vi "Display Info.vi"(7 "Layout ref":refnum<vi>, 8 "error in (no error)":errorcluster, 9 "Modify (F) /Add [T]":bool, 10 "Names in use":string[](array[string]), 11 "DDS in":refnum<class "DDS.lvclass">) -> (0 "error out":errorcluster, 1 "Names in use out":string[](array[string]), 2 "Changes Made?":bool, 3 "DDS out":refnum<class "DDS.lvclass">)   [LabVIEW 2013, in "DDS.lvclass"]
uses:
  DDS.lvclass
  TypeDefs/DigitalColumnAppearCluster.ctl
  TypeDefs/ColumnAppearCluster.ctl
  DDS.lvclass/DDS.ctl
  ColumnVIs/Column/Column.lvclass
panel:
  out "Col. Appear. Labels":string[](array[string])
  in  "Column appearance":T1[](array[typedef])
  in  "Sweep Dir. Appearance":T2={"Column Name"="", "Width"=18, "Bkgd"=[1985280, 6618880, 14090026], "Text"=[16448250, 0, 0]}
  in  "Cancel":bool
  in  "Device Description":string
  in  "DDS config":T3={"PB trig / Sequence"=FALSE, "Sweeps"=FALSE, "Amp Lock"=FALSE, "Master Trig. Line"=4, "USB Chan. name"=""}
  in  "Done":bool
  in  "Name":string
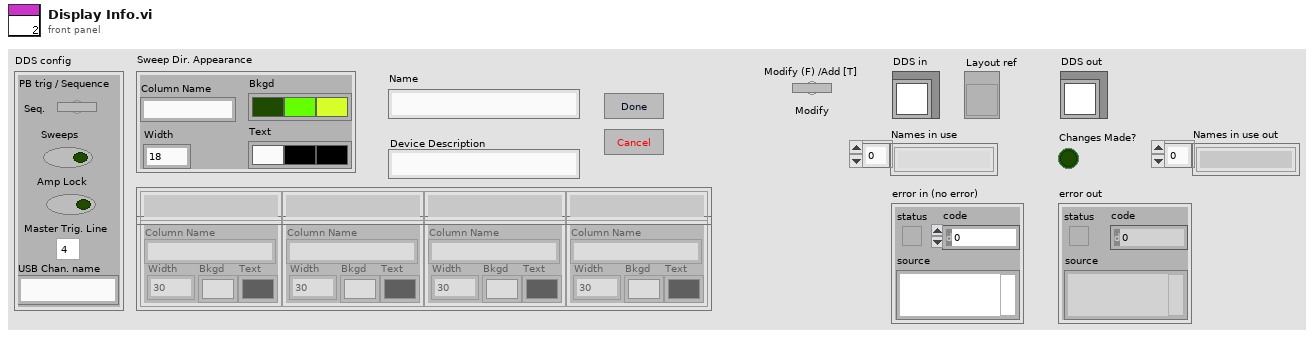
[diagram p1: front panel]
types:
  T1 = typedef "ColumnAppearCluster.ctl" = cluster{"Column Name":string, "Width":u32, "Bkgd":u32[], "Text":u32[]}
  T2 = typedef "DigitalColumnAppearCluster.ctl" = cluster{"Column Name":string, "Width":u32, "Bkgd":u32[], "Text":u32[]}
  T3 = cluster{"PB trig / Sequence":bool, "Sweeps":bool, "Amp Lock":bool, "Master Trig. Line":u16, "USB Chan. name":string}
  T4 = enum8{"Enabled", "Disabled", "Disabled and Grayed Out"}
  T5 = cluster{"Sweeps":bool, "PB trig / Sequence":bool, "Amp Lock":bool, "Firmware Ver":dbl}
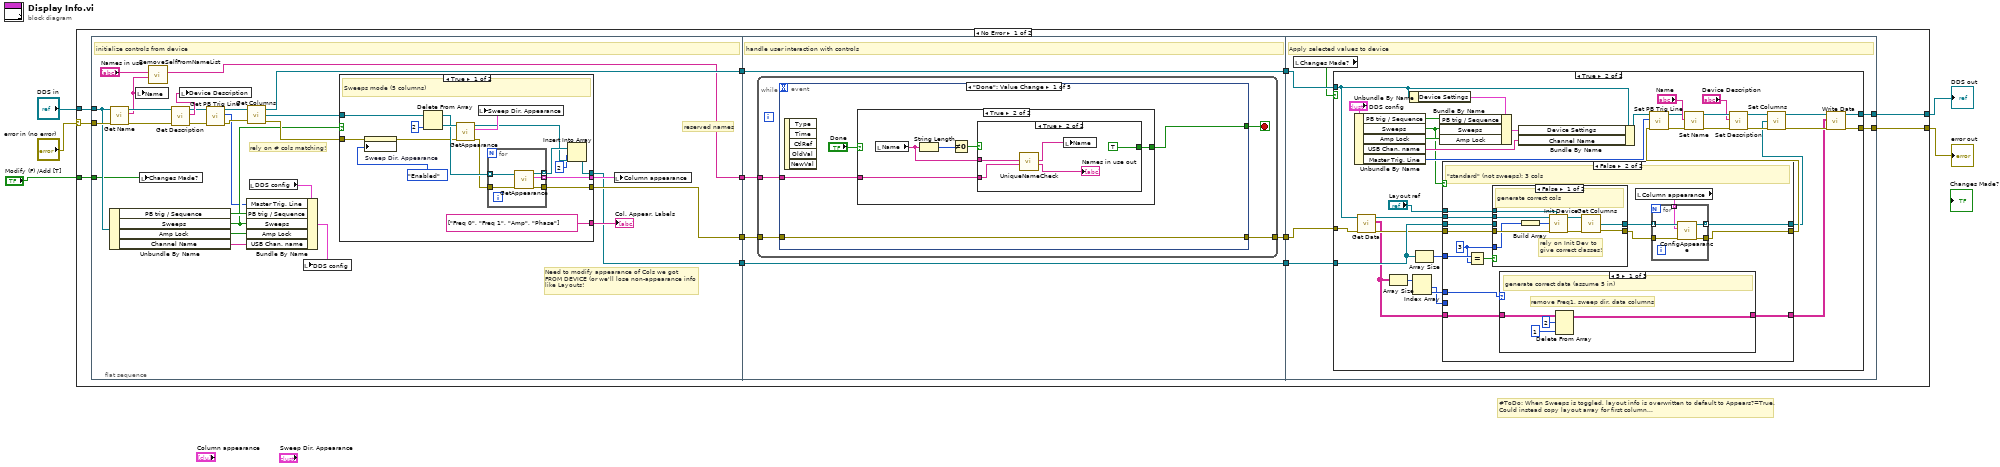
[diagram p0: block diagram]
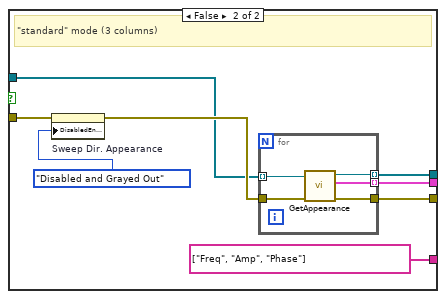
[diagram p2: hidden frame]
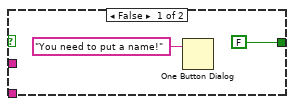
[diagram p4: hidden frame]
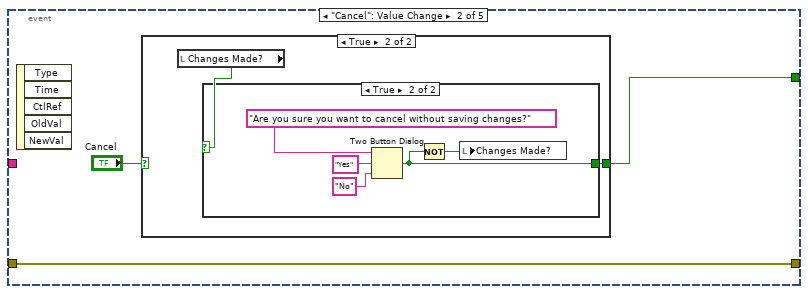
[diagram p5: hidden frame]
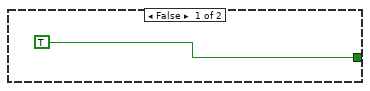
[diagram p7: hidden frame]
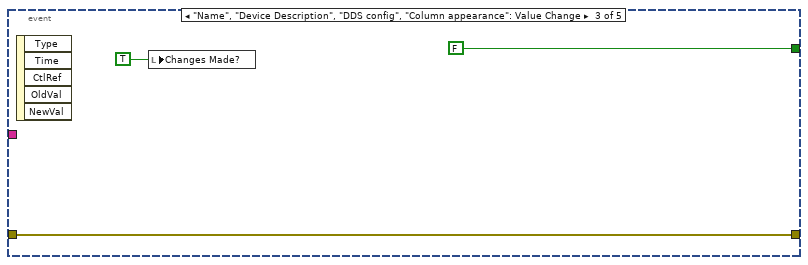
[diagram p8: hidden frame]
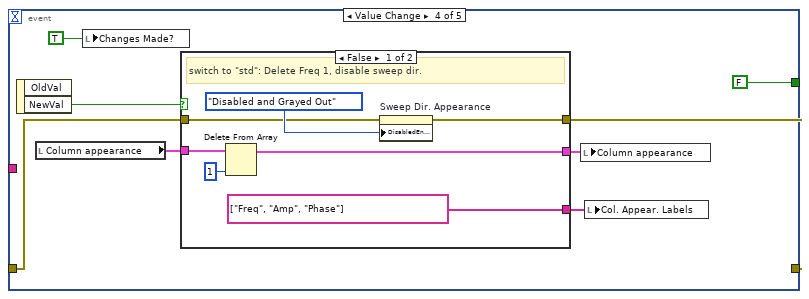
[diagram p9: hidden frame]
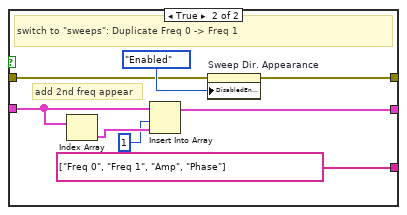
[diagram p10: hidden frame]
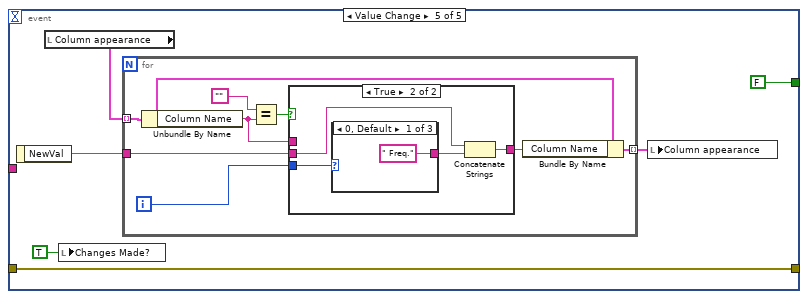
[diagram p11: hidden frame]
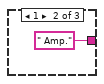
[diagram p13: hidden frame]
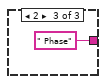
[diagram p14: hidden frame]
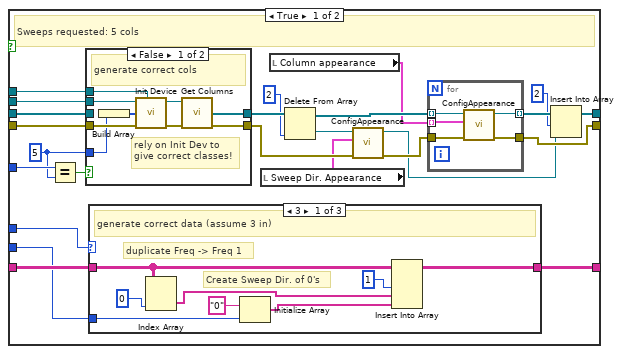
[diagram p16: hidden frame]
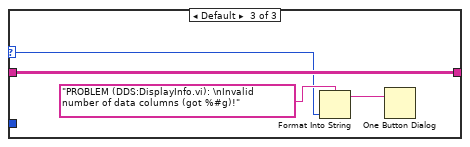
[diagram p18: hidden frame]
diagram:
  # "#ToDo: When Sweeps is toggled, layout info is overwritten to default to Appears?=True.\nCould instead copy layout array for first column..."
  n1 = case shown="No Error" "error in (no error)" {
    selector: "error in (no error)" -> [w14 w302]
    tunnel: [w11 w302] -> w4
    tunnel: "DDS in" -> [w8 w301]
    tunnel: [w17 w301] -> w2
    tunnel: "Modify (F) /Add [T]" -> [w7 _]
    frame No Error {
      n2 = flat-sequence {
        tunnel: [w43] -> w16
        tunnel: w14 -> [w30]
        tunnel: [w29] -> w13
        tunnel: [w28] -> w10
        tunnel: w8 -> [w22]
        tunnel: w7 -> [w21]
        tunnel: [w18] -> w6
        tunnel: w16 -> [w83]
        tunnel: [w83] -> w15
        tunnel: w13 -> [w82]
        tunnel: [w81] -> w12
        tunnel: w10 -> [w80]
        tunnel: [w80] -> w9
        tunnel: w6 -> [w79]
        tunnel: [w170] -> w17
        tunnel: w15 -> [w169]
        tunnel: w12 -> [w165]
        tunnel: [w167] -> w11
        tunnel: w9 -> [w166]
        frame #0 {
          # "reserved names"
          # "Need to modify appearance of Cols we got\nFROM DEVICE (or we'll lose non-appearance info\nlike Layouts!"
          # "rely on # cols matching!"
          # "initialize controls from device"
          n3 = Unbundle By Name(w22) -> ("PB trig / Sequence"=w27:bool, "Sweeps"=w26:bool, "Amp Lock"=w25:bool, "Channel Name"=w40:string)
          n4 = call-dynamic "Get Name.vi"("error in (no error)"=w30, "Device in"=w22) -> ("error out"=w37:errorcluster, "Name"=w19:string, "Device out"=w39:refnum<class "DDS.lvclass">)  [unwired: 7 in]
          n5 = local write "Name"(w19) -> ()
          n6 = local write "Changes Made?"(w21) -> ()
          n7 = call "RemoveSelfFromNameList.vi"("self Name"=w19, "Names in use"="Names in use") -> ("Reserved Names"=w18:string[])  [unwired: 9 in]
          n8 = call-dynamic "Get Description.vi"("error in (no error)"=w37, "Device in"=w39) -> ("error out"=w36:errorcluster, "Device Description"=w44:string, "Device out"=w38:refnum<class "DDS.lvclass">)  [unwired: 7 in]
          n9 = local write "Device Description"(w44) -> ()
          n10 = call-dynamic "Get PB Trig Line.vi"("error in (no error)"=w36, "Device in"=w38) -> ("error out"=w34:errorcluster, "PB Trigger Line"=w24:u16, "Device out"=w35:refnum<class "DDS.lvclass">)  [unwired: 7 in]
          n11 = call-dynamic "Get Columns.vi"("Device in"=w35, "error in (no error)"=w34) -> ("Device out"=w43:refnum<class "DDS.lvclass">, "Columns"=w23:refnum<class "Column.lvclass">[], "error out"=w33:errorcluster)
          n12 = local read "DDS config"() -> (w42:T3)
          n13 = Bundle By Name(cluster=w42, "Master Trig. Line"=w24, "PB trig / Sequence"=w27, "Sweeps"=w26, "Amp Lock"=w25, "USB Chan. name"=w40) -> (w41:T3)
          n14 = local write "DDS config"(w41) -> ()
          n15 = case shown="True" w26 {
            tunnel: w33 -> [w52 w71]
            tunnel: w23 -> [w57 w68]
            tunnel: [string[] ["Freq 0", "Freq 1", "Amp", "Phase"] ("Col. Appear. Labels") string[] ["Freq", "Amp", "Phase"] ("Col. Appear. Labels")] -> w32
            tunnel: [w53 w72] -> w31
            tunnel: [w49 w67] -> w29
            tunnel: [w47 w66] -> w28
            frame True {
              # "Sweeps mode (5 columns)"
              n16 = property on="Sweep Dir. Appearance" class="Clust (strict)"(error in=w52, "DisabledEnum"=T4."Enabled" ("Disabled")) -> (error out=w51:errorcluster)  [unwired: 1 in, 1 out]
              n17 = Delete From Array "Delete From Array"(array=w57, index=2) -> (deleted portion=w59:refnum<class "Column.lvclass">, array with subset deleted=w56:refnum<class "Column.lvclass">[])  [unwired: 1 in]
              n18 = call "GetAppearance.vi"("error in (no error)"=w51, "Column in"=w59) -> ("error out"=w55:errorcluster, "Column Appearance"=w58:T1, "Column out"=w46:refnum<class "Column.lvclass">)  [unwired: 7 in]
              n19 = local write "Sweep Dir. Appearance"(w58) -> ()
              n20 = for {
                tunnel: w56 -> [w65] mode=indexing
                tunnel: w55 -> [w64]
                tunnel: [w63] -> w53 mode=indexing
                tunnel: [w62] -> w49
                tunnel: [w61] -> w48 mode=indexing
                n21 = call "GetAppearance.vi"("error in (no error)"=w64, "Column in"=w65) -> ("error out"=w62:errorcluster, "Column Appearance"=w63:T1, "Column out"=w61:refnum<class "Column.lvclass">)  [unwired: 7 in]
              }
              n22 = Insert Into Array(array=w48, index=2, new element=w46) -> (w47:refnum<class "Column.lvclass">[])
            }
            frame False {
              # "\"standard\" mode (3 columns)"
              n23 = property on="Sweep Dir. Appearance" class="Clust (strict)"(error in=w71, "DisabledEnum"=T4."Disabled and Grayed Out" ("Disabled")) -> (error out=w69:errorcluster)  [unwired: 1 in, 1 out]
              n24 = for {
                tunnel: w68 -> [w78] mode=indexing
                tunnel: w69 -> [w77]
                tunnel: [w76] -> w72 mode=indexing
                tunnel: [w75] -> w67
                tunnel: [w74] -> w66 mode=indexing
                n25 = call "GetAppearance.vi"("error in (no error)"=w77, "Column in"=w78) -> ("error out"=w75:errorcluster, "Column Appearance"=w76:T1, "Column out"=w74:refnum<class "Column.lvclass">)  [unwired: 7 in]
              }
            }
          }
          "Col. Appear. Labels" <- w32
          n26 = local write "Column appearance"(w31) -> ()
        }
        frame #1 {
          # "handle user interaction with controls"
          n27 = while {
            tunnel: w82 -> [w86]
            tunnel: [w85] -> w81
            tunnel: w79 -> [w84]
            stop <- w87 stop-if-true
            n28 = event shown="[0] \"Done\": Value Change" {
              selector: _ -> [_ _ _ _ _]
              dyn-events: _ -> [_ _ _ _ _]
              timeout: _ -> [_ _ _ _ _]
              tunnel: [w90 w106 FALSE ("T button?") FALSE ("T button?") FALSE ("T button?")] -> w87
              tunnel: w86 -> [w89 w105 w117 w121 w143]
              tunnel: [w89 w105 w117 w120 w143] -> w85
              tunnel: w84 -> [w88 _ _ _ _]
              event "Done": Value Change {
                n29 = event-data() -> ()  [unwired: 1 in, 5 out]
                n30 = case shown="True" "Done" {
                  selector: "Done" -> [w92 _]
                  tunnel: [w92 w95] -> w90
                  tunnel: w88 -> [_ w93]
                  frame False {
                  }
                  frame True {
                    n31 = local read "Name"() -> (w94:string)
                    n32 = String Length(string=w94) -> (length=w97:i32)
                    n33 = Not Equal To 0?(x=w97) -> (x != 0?=w96:bool)
                    n34 = case shown="True" w96 {
                      tunnel: [FALSE TRUE] -> w95
                      tunnel: w94 -> [_ w103]
                      tunnel: w93 -> [_ w102]
                      frame False {
                        n35 = One Button Dialog(message="You need to put a name!") -> ()  [unwired: 1 in, 1 out]
                      }
                      frame True {
                        n36 = call "UniqueNameCheck.vi"("Names in use"=w102, "Device Name"=w103) -> ("Names in use out"=→"Names in use out":string[], "Unique name"=w101:string)  [unwired: 8 in]
                        n37 = local write "Name"(w101) -> ()
                      }
                    }
                  }
                }
              }
              event "Cancel": Value Change {
                n38 = event-data() -> ()  [unwired: 1 in, 5 out]
                n39 = case shown="True" "Cancel" {
                  selector: "Cancel" -> [w108 _]
                  tunnel: [w108 w110] -> w106
                  frame False {
                  }
                  frame True {
                    n40 = local read "Changes Made?"() -> (w109:bool)
                    n41 = case shown="True" w109 {
                      tunnel: [TRUE w113] -> w110
                      frame False {
                      }
                      frame True {
                        n42 = Two Button Dialog(message="Are you sure you want to cancel without saving changes?", 1:"No", 2:"Yes") -> (T button?=w113:bool)
                        n43 = Not(x=w113) -> (.not. x?=w112:bool)
                        n44 = local write "Changes Made?"(w112) -> ()
                      }
                    }
                  }
                }
              }
              event "Name", "Device Description", "DDS config", "Column appearance": Value Change {
                n45 = event-data() -> ()  [unwired: 1 in, 5 out]
                n46 = local write "Changes Made?"(TRUE) -> ()
              }
              event "DDS config.Sweeps": Value Change {
                n47 = event-data() -> ("NewVal"=w126:bool)  [unwired: 1 in, 1 out]
                n48 = local read "Column appearance"() -> (w124:T1[])
                n49 = local write "Changes Made?"(TRUE ("Changes Made?")) -> ()
                n50 = case shown="False" w126 {
                  tunnel: [string[] ["Freq", "Amp", "Phase"] ("Col. Appear. Labels") string[] ["Freq 0", "Freq 1", "Amp", "Phase"] ("Col. Appear. Labels")] -> w125
                  tunnel: w124 -> [w132 w139]
                  tunnel: [w130 w140] -> w123
                  tunnel: w121 -> [w129 w135]
                  tunnel: [w128 w136] -> w120
                  frame False {
                    # "switch to \"std\": Delete Freq 1, disable sweep dir."
                    n51 = Delete From Array "Delete From Array"(array=w132, index=1) -> (array with subset deleted=w130:T1[])  [unwired: 1 in, 1 out]
                    n52 = property on="Sweep Dir. Appearance" class="Clust (strict)"(error in=w129, "DisabledEnum"=T4."Disabled and Grayed Out" ("Disabled")) -> (error out=w128:errorcluster)  [unwired: 1 in, 1 out]
                  }
                  frame True {
                    # "add 2nd freq appear"
                    # "switch to \"sweeps\": Duplicate Freq 0 -> Freq 1"
                    n53 = Index Array(array=w139) -> (element=w138:T1)  [unwired: 1 in]
                    n54 = Insert Into Array "Insert Into Array"(array=w139, index=1, new element=w138) -> (w140:T1[])
                    n55 = property on="Sweep Dir. Appearance" class="Clust (strict)"(error in=w135, "DisabledEnum"=T4."Enabled" ("Disabled")) -> (error out=w136:errorcluster)  [unwired: 1 in, 1 out]
                  }
                }
                n56 = local write "Column appearance"(w123) -> ()
                n57 = local write "Col. Appear. Labels"(w125) -> ()
              }
              event "DDS config.USB Chan. name": Value Change {
                n58 = event-data() -> ("NewVal"=w147:string)  [unwired: 1 in]
                n59 = local read "Column appearance"() -> (w145:T1[])
                n60 = local write "Changes Made?"(TRUE) -> ()
                n61 = for {
                  tunnel: w145 -> [w152] mode=indexing
                  tunnel: [w153] -> w144 mode=indexing
                  tunnel: w147 -> [w151]
                  i -> [w155]
                  n62 = Unbundle By Name(w152) -> ("Column Name"=w149:string)
                  n63 = Equal?(x="", y=w149) -> (x = y?=w154:bool)
                  n64 = case shown="True" w154 {
                    tunnel: w151 -> [_ w158]
                    tunnel: [w157 w159] -> w156
                    tunnel: w155 -> [_ w161]
                    tunnel: w149 -> [w157 _]
                    frame False {
                    }
                    frame True {
                      n65 = case shown="0, Default" w161 {
                        tunnel: [" Freq." " Amp." " Phase"] -> w160
                        frame 0, Default {
                        }
                        frame 1 {
                        }
                        frame 2 {
                        }
                      }
                      n66 = Concatenate Strings(w158, w160) -> (w159:string)
                    }
                  }
                  n67 = Bundle By Name(cluster=w152, "Column Name"=w156) -> (w153:T1)
                }
                n68 = local write "Column appearance"(w144) -> ()
              }
            }
          }
        }
        frame #2 {
          # "Apply selected values to device"
          n69 = local read "Changes Made?"() -> (w168:bool)
          n70 = case shown="True" w168 {
            tunnel: [w172 w178] -> w170
            tunnel: w169 -> [w172 w185]
            tunnel: [w171 w176] -> w167
            tunnel: w166 -> [_ w189]
            tunnel: w165 -> [w171 w184]
            frame False {
            }
            frame True {
              n71 = Unbundle By Name("DDS config") -> ("PB trig / Sequence"=w202:bool, "Sweeps"=w192:bool, "Amp Lock"=w201:bool, "USB Chan. name"=w199:string, "Master Trig. Line"=w198:u16)
              n72 = call-dynamic "Get Data.vi"("error in (no error)"=w184, "Device in"=w185) -> ("error out"=w182:errorcluster, "Table Indicator"=w181:string[][], "Device out"=w183:refnum<class "DDS.lvclass">)  [unwired: 6 in]
              n73 = Array Size(array=w181) -> (size(s)=w180:i32[])
              n74 = Unbundle By Name(w185) -> ("Device Settings"=w203:T5)
              n75 = Index Array(array=w180) -> (element #1=w173:i32, element #2=w174:i32)  [unwired: 2 in]
              n76 = Array Size(array=w189) -> (size(s)=w191:i32)
              n77 = Bundle By Name(cluster=w203, "PB trig / Sequence"=w202, "Sweeps"=w192, "Amp Lock"=w201) -> (w200:T5)
              n78 = case shown="False" w192 {
                tunnel: w191 -> [w231 w275]
                tunnel: w189 -> [w229 w274]
                tunnel: [w217 w271] -> w188
                tunnel: [w220 w272] -> w187
                tunnel: "Layout ref" -> [w215 w267]
                tunnel: w183 -> [w214 w266]
                tunnel: w182 -> [w213 w265]
                tunnel: w181 -> [w211 w264]
                tunnel: w174 -> [w209 w262]
                tunnel: [w212 w263] -> w175
                tunnel: w173 -> [w210 _]
                frame True {
                  w208 = 5 ("index")
                  # "Sweeps requested: 5 cols"
                  n79 = Equal?(x=w231, y=w208) -> (x = y?=w230:bool)
                  n80 = case shown="False" w230 {
                    tunnel: w214 -> [w258 _]
                    tunnel: [w255 w260] -> w228
                    tunnel: w229 -> [_ w260]
                    tunnel: [w254 w259] -> w223
                    tunnel: w213 -> [w253 w259]
                    tunnel: w215 -> [w252 _]
                    tunnel: w208 -> [w250 _]
                    frame False {
                      # "rely on Init Dev to \ngive correct classes!"
                      # "generate correct cols"
                      n81 = Build Array(w250) -> (w251:i32[])
                      n82 = call-dynamic "Init Device.vi"("Layout Ref"=w252, "error in (no error)"=w253, "Chan# Array"=w251, "DDS in"=w258) -> ("error out"=w256:errorcluster, "DDS out"=w257:refnum<class "DDS.lvclass">)  [unwired: 6 in]
                      n83 = call-dynamic "Get Columns.vi"("Device in"=w257, "error in (no error)"=w256) -> ("Columns"=w255:refnum<class "Column.lvclass">[], "error out"=w254:errorcluster)  [unwired: 1 out]
                    }
                    frame True {
                      # "correct # cols"
                    }
                  }
                  n84 = case shown="3" w209 {
                    selector: w209 -> [_ _ w242]
                    tunnel: [w238 w240 w244] -> w212
                    tunnel: w211 -> [w237 w240 w244]
                    tunnel: w210 -> [w234 _ _]
                    frame 3 {
                      # "Create Sweep Dir. of 0's"
                      # "duplicate Freq -> Freq 1"
                      # "generate correct data (assume 3 in)"
                      n85 = Index Array(array=w237, index (col)=0 ("disabled index (col)")) -> (element=w232:string[])  [unwired: 1 in]
                      n86 = Initialize Array("0", w234) -> (w233:string[])
                      n87 = Insert Into Array(array=w237, index (col)=1 ("disabled index (col)"), new element #1=w232, new element #2=w233) -> (w238:string[][])  [unwired: 1 in]
                    }
                    frame 0, 5 {
                      # "If length is 0, Default Data will take care within Add device."
                      # "correct data size"
                    }
                    frame Default {
                      n88 = Format Into String(format string="PROBLEM (DDS:DisplayInfo.vi): \nInvalid number of data columns (got %#g)!" ("message"), w242) -> (resulting string=w241:string)  [unwired: 2 in, 1 out]
                      n89 = One Button Dialog(message=w241) -> ()  [unwired: 1 in, 1 out]
                    }
                  }
                  n90 = local read "Sweep Dir. Appearance"() -> (w218:T2)
                  n91 = local read "Column appearance"() -> (w225:T1[])
                  n92 = Delete From Array(array=w228, index=2) -> (deleted portion=w224:refnum<class "Column.lvclass">, array with subset deleted=w226:refnum<class "Column.lvclass">[])  [unwired: 1 in]
                  n93 = call "ConfigAppearance.vi"("error in (no error)"=w223, "Column Appearance"=w218, "Column in"=w224) -> ("error out"=w222:errorcluster, "Column out"=w216:refnum<class "Column.lvclass">)  [unwired: 7 in]
                  n94 = for {
                    tunnel: w226 -> [w249] mode=indexing
                    tunnel: [w248] -> w221 mode=indexing
                    tunnel: [w247] -> w217
                    tunnel: w222 -> [w246]
                    tunnel: w225 -> [w245] mode=indexing
                    n95 = call "ConfigAppearance.vi"("error in (no error)"=w246, "Column Appearance"=w245, "Column in"=w249) -> ("error out"=w247:errorcluster, "Column out"=w248:refnum<class "Column.lvclass">)  [unwired: 7 in]
                  }
                  n96 = Insert Into Array(array=w221, index=2, new element=w216) -> (w220:refnum<class "Column.lvclass">[])
                }
                frame False {
                  w261 = 3 ("index")
                  # "\"standard\" (not sweeps): 3 cols"
                  n97 = Equal?(x=w275, y=w261) -> (x = y?=w268:bool)
                  n98 = case shown="False" w268 {
                    tunnel: [w292 w300] -> w273
                    tunnel: w274 -> [_ w300]
                    tunnel: [w296 w299] -> w270
                    tunnel: w267 -> [w295 _]
                    tunnel: w266 -> [w294 _]
                    tunnel: w265 -> [w293 w299]
                    tunnel: w261 -> [w290 _]
                    frame False {
                      # "rely on Init Dev to \ngive correct classes!"
                      # "generate correct cols"
                      n99 = Build Array(w290) -> (w291:i32[])
                      n100 = call-dynamic "Init Device.vi"("Layout Ref"=w295, "error in (no error)"=w293, "Chan# Array"=w291, "DDS in"=w294) -> ("error out"=w297:errorcluster, "DDS out"=w298:refnum<class "DDS.lvclass">)  [unwired: 6 in]
                      n101 = call-dynamic "Get Columns.vi"("Device in"=w298, "error in (no error)"=w297) -> ("Columns"=w292:refnum<class "Column.lvclass">[], "error out"=w296:errorcluster)  [unwired: 1 out]
                    }
                    frame True {
                      # "correct # cols"
                    }
                  }
                  n102 = case shown="5" w262 {
                    selector: w262 -> [_ _ w283]
                    tunnel: [w276 w280 w284] -> w263
                    tunnel: w264 -> [w279 w280 w284]
                    frame 5 {
                      # "remove Freq1, sweep dir. data columns"
                      # "generate correct data (assume 5 in)"
                      n103 = Delete From Array(array=w279, length=2, index (col)=1 ("disabled index (col)")) -> (array with subset deleted=w276:string[][])  [unwired: 1 in, 1 out]
                    }
                    frame 0, 3 {
                      # "If length is 0, Default Data will take care next, within Add device."
                      # "correct data size"
                    }
                    frame Default {
                      n104 = Format Into String(format string="PROBLEM (DDS:DisplayInfo.vi): \nInvalid number of data columns (got %#g)!" ("message"), w283) -> (resulting string=w281:string)  [unwired: 2 in, 1 out]
                      n105 = One Button Dialog(message=w281) -> ()  [unwired: 1 in, 1 out]
                    }
                  }
                  n106 = local read "Column appearance"() -> (w269:T1[])
                  n107 = for {
                    tunnel: w273 -> [w289] mode=indexing
                    tunnel: [w288] -> w272 mode=indexing
                    tunnel: [w287] -> w271
                    tunnel: w270 -> [w286]
                    tunnel: w269 -> [w285] mode=indexing
                    n108 = call "ConfigAppearance.vi"("error in (no error)"=w286, "Column Appearance"=w285, "Column in"=w289) -> ("error out"=w287:errorcluster, "Column out"=w288:refnum<class "Column.lvclass">)  [unwired: 7 in]
                  }
                }
              }
              n109 = Bundle By Name(cluster=w185, "Device Settings"=w200, "Channel Name"=w199) -> (w190:refnum<class "DDS.lvclass">)
              n110 = call-dynamic "Set PB Trig Line.vi"("error in (no error)"=w188, "PB Trigger Line"=w198, "Device in"=w190) -> ("error out"=w196:errorcluster, "Device out"=w197:refnum<class "DDS.lvclass">)  [unwired: 7 in]
              n111 = call-dynamic "Set Name.vi"("error in (no error)"=w196, "Name"="Name", "Device in"=w197) -> ("error out"=w195:errorcluster, "Device out"=w207:refnum<class "DDS.lvclass">)  [unwired: 7 in]
              n112 = call-dynamic "Set Description.vi"("error in (no error)"=w195, "Device Description"="Device Description", "Device in"=w207) -> ("error out"=w193:errorcluster, "Device out"=w194:refnum<class "DDS.lvclass">)  [unwired: 7 in]
              n113 = call-dynamic "Set Columns.vi"("error in (no error)"=w193, "Columns in"=w187, "DDS in"=w194) -> ("error out"=w177:errorcluster, "DDS out"=w179:refnum<class "DDS.lvclass">)  [unwired: 1 in]
              n114 = call-dynamic "Write Data.vi"("error in (no error)"=w177, "Data"=w175, "Device in"=w179) -> ("error out"=w176:errorcluster, "Device Out"=w178:refnum<class "DDS.lvclass">)  [unwired: 7 in]
            }
          }
        }
      }
    }
    frame Error {
    }
  }
  "error out" <- w4
  "DDS out" <- w2
